vi "VeriStand Example.vi"() -> ()   [LabVIEW 2015]
uses:
  VeriStand FPGA Generation Wizard/Source/SubModules/FPGA Addon Speciality IO/Source/Types/PWM.Measure.Digital.Measurement.ctl
  VeriStand FPGA Generation Wizard/Source/SubModules/FPGA Addon Speciality IO/Source/Types/PWM.Generate.Digital.Settings.ctl
  VeriStand FPGA Generation Wizard/Source/SubModules/FPGA Addon Speciality IO/Source/Types/PWM.Measure.Analog.Measurement.ctl
  VeriStand FPGA Generation Wizard/Source/SubModules/FPGA Addon Speciality IO/Source/Types/PWM.Measure.Digital.Settings.ctl
  VeriStand FPGA Generation Wizard/Source/SubModules/FPGA Addon Speciality IO/Source/Types/PWM.Measure.Analog.Settings.ctl
  VeriStand FPGA Generation Wizard/Source/SubModules/FPGA Addon Speciality IO/Source/Types/Sine.Generate.Settings.ctl
  VeriStand FPGA Generation Wizard/Source/SubModules/FPGA Addon Speciality IO/Source/Types/Static.Generate.Digital.Settings.ctl
  VeriStand FPGA Generation Wizard/Source/SubModules/FPGA Addon Speciality IO/Source/Types/Static.Measure.Digital.Settings.ctl
  VeriStand FPGA Generation Wizard/Source/SubModules/FPGA Addon Speciality IO/Source/Types/Static.Measure.Digital.Measurement.ctl
  VeriStand FPGA Generation Wizard/Source/SubModules/FPGA Addon Speciality IO/Source/Types/WSS.Generate.Digital.Settings.ctl
  VeriStand FPGA Generation Wizard/Source/SubModules/FPGA Addon Speciality IO/Source/Types/QuadratureEncoder.Measure.Digital.Measurement.ctl
  VeriStand FPGA Generation Wizard/Source/SubModules/FPGA Addon Speciality IO/Source/Types/QuadratureEncoder.Measure.Digital.Settings.ctl
  <vilib>/Platform/TimedLoop/XDataNode/timing_clust.ctl
  <vilib>/Platform/TimedLoop/XDataNode/nitl_modes.ctl
  <vilib>/Platform/TimedLoop/XDataNode/wakeup.ctl
  <vilib>/rvi/Emulation/niFpgaGetClockAttributes.vi
  <vilib>/rvi/Emulation/niFpgaSctlEmulationGetInTimedLoop.vi
  <vilib>/rvi/Emulation/niFpgaEmulationReportErrorSimple.vi
  <vilib>/rvi/Emulation/niFpgaCriticalErrorInLSC.vi
  <vilib>/Platform/TimedLoop/XDataNode/XDataNode.xnode
  VeriStand FPGA Generation Wizard/Source/SubModules/FPGA Addon Speciality IO/Source/Speciality FPGA IO.lvlib
  <vilib>/Platform/TimedLoop/XDataNode/XDNodeRunTimeDep.lvlib
panel:
  in  "Measure.Digital.Ch5.QuadEncoder.Settings":T1={"DIRECTION"=0, "RESET VALUE"=0, "A RESET STATE"=TRUE, "B RESET STATE"=TRUE, "Z RESET STATE"=TRUE}
  in  "Z":bool
  in  "B":bool
  in  "A":bool
  out "Measurement.Digital.Ch5":T2
  out "Bit1":bool
  out "Bit0":bool
  in  "Generate.Digital.Ch4.WSS.Settings":T3={"ACTIVE EDGE"=TRUE, "ACTIVE TICKS"=0, "INACTIVE TICKS"=0, "DATA"=0, "SENSOR TYPE"=0}
  in  "Generate.Digital.Ch3.Internal.Settings":T4={"ACTIVE EDGE"=TRUE, "OUTPUT"=FALSE}
  in  "Measure.Digital.Ch3.Internal.Settings":T5={"ACTIVE EDGE"=TRUE}
  out "Measure.Digital.Ch3":T6
  out "Measure.Digital.Ch2":T6
  in  "Measure.Digital.Ch2.Internal.Settings":T5={"ACTIVE EDGE"=TRUE}
  in  "Generate.Digital.Ch2.Internal.Settings":T4={"ACTIVE EDGE"=TRUE, "OUTPUT"=FALSE}
  out "Analog.Generation.Ticks":u32=10 caption="Count(uSec)"
  in  "Generate.Sine.Ch1.Settings":T7
  in  "Generate.Sine.Ch0.Settings":T7
  in  "Sine":bool=TRUE
  in  "Measure.Analog.Ch1.Settings":T8={"ACTIVE EDGE"=FALSE, "TIMEOUT"=40000000, "THRESHOLD"=95.0}
  in  "Measure.Analog.Ch0.Settings":T8={"ACTIVE EDGE"=TRUE, "TIMEOUT"=40000000, "THRESHOLD"=0.0}
  in  "Measure.Digital.Ch1.Settings":T9={"ACTIVE EDGE"=FALSE, "TIMEOUT"=40000000}
  in  "Measure.Digital.Ch0.Settings":T9={"ACTIVE EDGE"=TRUE, "TIMEOUT"=40000000}
  out "Measure.Analog.Ch1":T10={"ACTIVE TICKS"=90, "INACTIVE TICKS"=10, "ACQ TICKS"=400, "ACTIVE VOLTAGE"=-6.998723030090332, "INACTIVE VOLTAGE"=6.998509407043457}
  out "Measure.Analog.Ch0":T10={"ACTIVE TICKS"=10, "INACTIVE TICKS"=10, "ACQ TICKS"=400, "ACTIVE VOLTAGE"=4.979251861572266, "INACTIVE VOLTAGE"=-4.979404449462891}
  in  "Generate.Digital.Ch1.Internal.Settings":T11={"ACTIVE EDGE"=FALSE, "ACTIVE TICKS"=60000000, "INACTIVE TICKS"=20000000}
  in  "Generate.Digital.Ch0.Internal.Settings":T11={"ACTIVE EDGE"=TRUE, "ACTIVE TICKS"=4000, "INACTIVE TICKS"=12000}
  out "Measure.Digital.Ch1":T12
  out "Measure.Digital.Ch0":T12={"ACTIVE TICKS"=4000, "INACTIVE TICKS"=12000, "ACQ TICKS"=1}
  in  "Analog.Generation.Ticks":u32=10 caption="Count(uSec)"
  # "98"
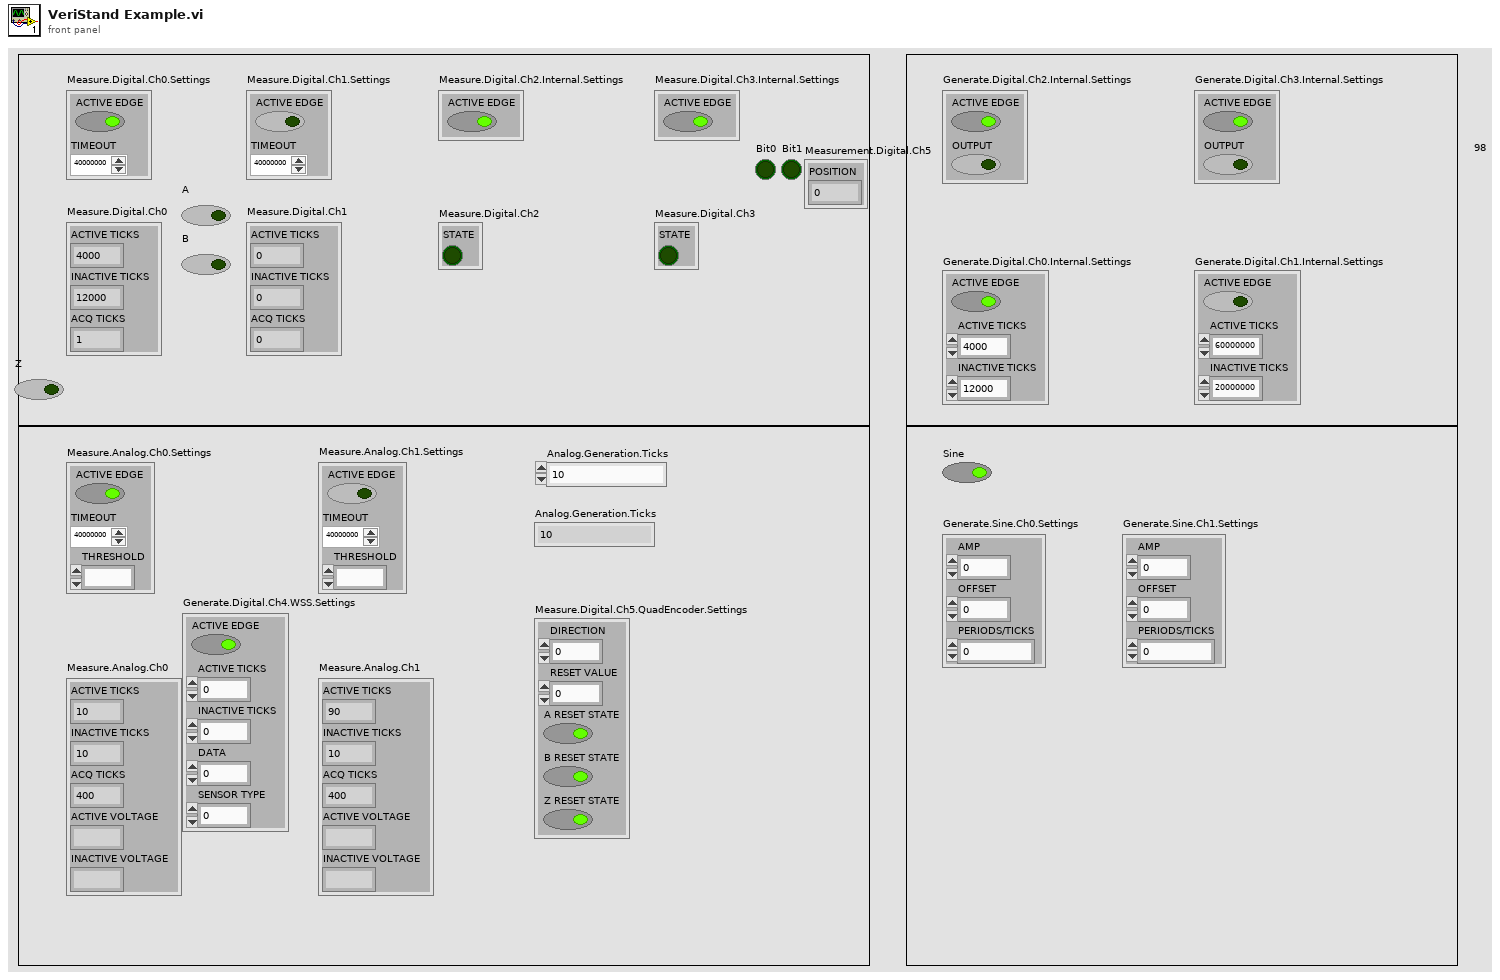
[diagram p1: front panel]
types:
  T1 = typedef "QuadratureEncoder.Measure.Digital.Settings.ctl" = cluster{"DIRECTION":u8, "RESET VALUE":i32, "A RESET STATE":bool, "B RESET STATE":bool, "Z RESET STATE":bool}
  T2 = typedef "QuadratureEncoder.Measure.Digital.Measurement.ctl" = cluster{"POSITION":i32}
  T3 = typedef "Speciality FPGA IO.lvlib/WSS.Generate.Digital.Settings.ctl" = cluster{"ACTIVE EDGE":bool, "ACTIVE TICKS":u32, "INACTIVE TICKS":u32, "DATA":u8, "SENSOR TYPE":u8}
  T4 = typedef "Speciality FPGA IO.lvlib/Static.Generate.Digital.Settings.ctl" = cluster{"ACTIVE EDGE":bool, "OUTPUT":bool}
  T5 = typedef "Speciality FPGA IO.lvlib/Static.Measure.Digital.Settings.ctl" = cluster{"ACTIVE EDGE":bool}
  T6 = typedef "Speciality FPGA IO.lvlib/Static.Measure.Digital.Measurement.ctl" = cluster{"STATE":bool}
  T7 = typedef "Speciality FPGA IO.lvlib/Sine.Generate.Settings.ctl" = cluster{"AMP":fxp<+/-,32,8>, "OFFSET":fxp<+/-,32,8>, "PERIODS/TICKS":fxp<+,32,0>}
  T8 = typedef "Speciality FPGA IO.lvlib/PWM.Measure.Analog.Settings.ctl" = cluster{"ACTIVE EDGE":bool, "TIMEOUT":u32, "THRESHOLD":fxp<+/-,32,8>}
  T9 = typedef "Speciality FPGA IO.lvlib/PWM.Measure.Digital.Settings.ctl" = cluster{"ACTIVE EDGE":bool, "TIMEOUT":u32}
  T10 = typedef "Speciality FPGA IO.lvlib/PWM.Measure.Analog.Measurement.ctl" = cluster{"ACTIVE TICKS":u32, "INACTIVE TICKS":u32, "ACQ TICKS":u32, "ACTIVE VOLTAGE":fxp<+/-,32,8>, "INACTIVE VOLTAGE":fxp<+/-,32,8>}
  T11 = typedef "Speciality FPGA IO.lvlib/PWM.Generate.Digital.Settings.ctl" = cluster{"ACTIVE EDGE":bool, "ACTIVE TICKS":u32, "INACTIVE TICKS":u32}
  T12 = typedef "Speciality FPGA IO.lvlib/PWM.Measure.Digital.Measurement.ctl" = cluster{"ACTIVE TICKS":u32, "INACTIVE TICKS":u32, "ACQ TICKS":u32}
  T13 = typedef "XDNodeRunTimeDep.lvlib/timing_clust.ctl" = cluster{"Expected End [f-1]":u64, "Actual End [f-1]":u64, "Finished Late? [f-1]":bool, "Expected End [i-1]":u64, "Actual End [i-1]":u64, "Finished Late? [i-1]":bool, "Expected Start [i]":u64, "Actual Start [i]":u64, "Expected Start [f]":u64, "Actual Start [f]":u64, "Source Name":string, "Structure Name":string, "Period":i64, "Deadline":i64, "Offset":i64, "Start":i64, "Priority":i32, "Timeout":i32, "Mode":T14, "Wakeup Reason":T15, "Error":errorcluster, "Source Type":string, "Secondary Source Type":string, "Global End Time":u64, "Global Start Time":u64, "Frame Duration":u64, "Iteration Duration":u64, "Assigned CPU":i32, "I/O Scan Engine Mode":u32}
  T14 = typedef "XDNodeRunTimeDep.lvlib/nitl_modes.ctl" = enum32{"No Change", "Process missed periods, maintain original phase", "Discard missed periods, maintain original phase", "Process missed periods, ignore original phase", "Discard missed periods, ignore original phase"}
  T15 = typedef "XDNodeRunTimeDep.lvlib/wakeup.ctl" = enum32{"Normal", "Aborted", "Asynchronous wakeup", "Timing source error", "Timed loop error", "Timeout"}
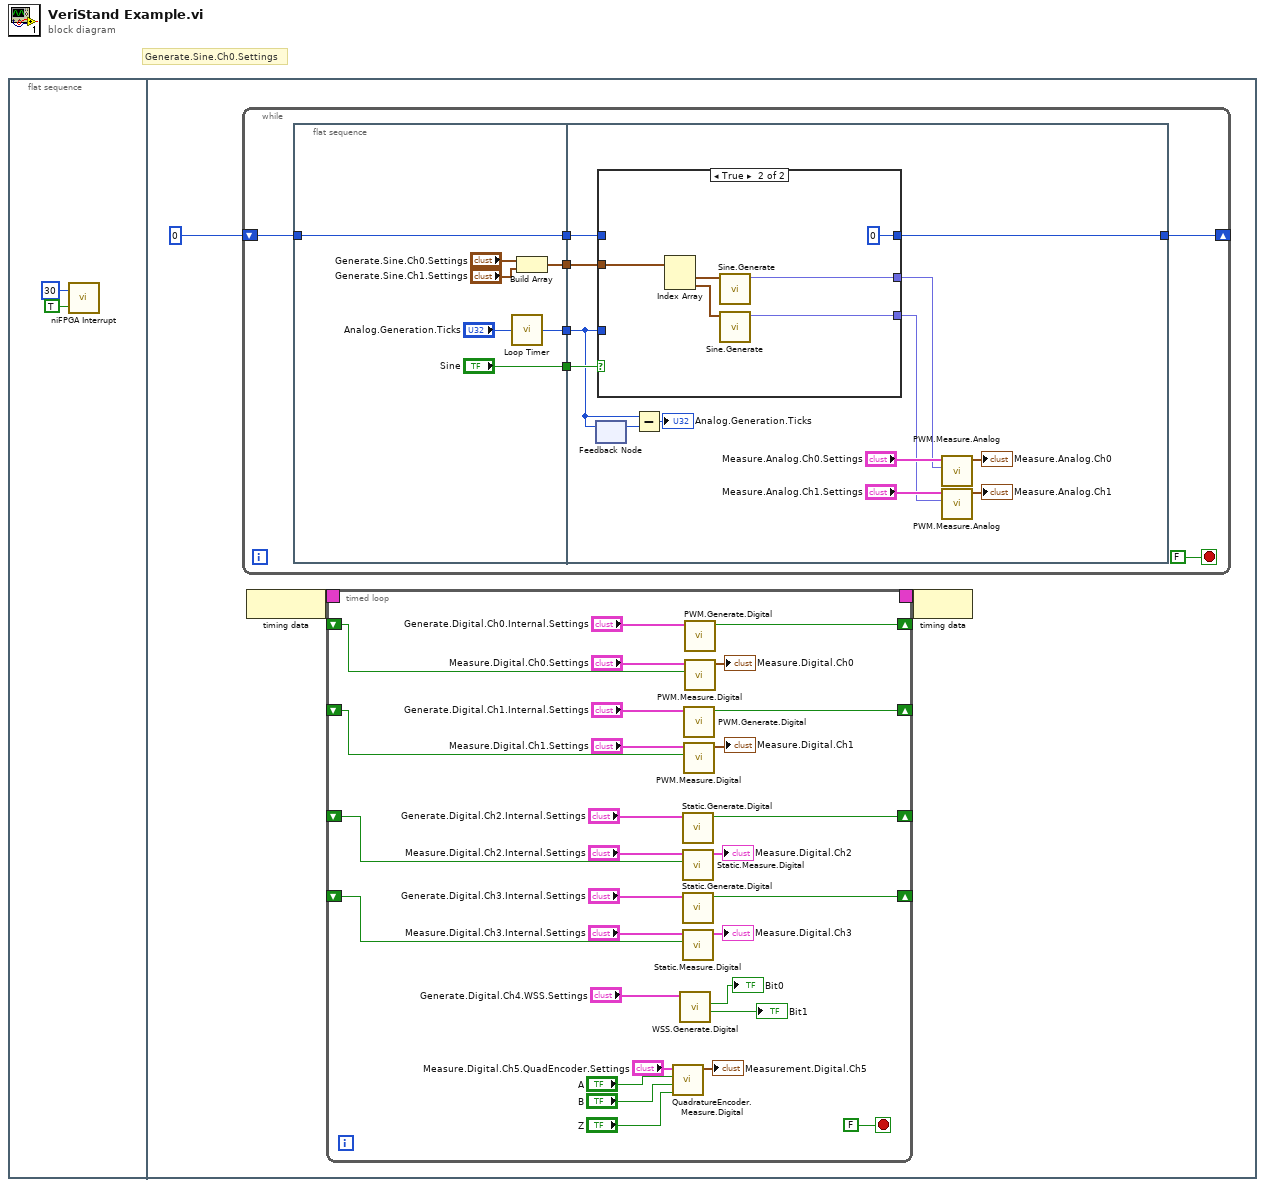
[diagram p0: block diagram]
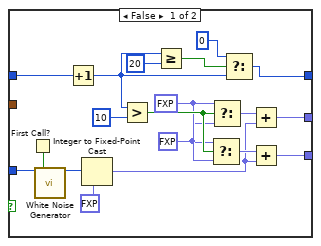
[diagram p2: hidden frame]
diagram:
  # "Generate.Sine.Ch0.Settings"
  n1 = flat-sequence {
    frame #0 {
      n2 = call <vilib>:"niFPGA Interrupt.vi"("Wait Until Cleared (F)"=TRUE, "IRQ Number (0)"=u8 30) -> ()  [unwired: 1 in]
    }
    frame #1 {
      n3 = while {
        shift-right: [w43] -> _
        shift-left: i16 0 -> [w44]
        stop <- FALSE stop-if-true
        n4 = flat-sequence {
          tunnel: [w51] -> w45
          tunnel: w44 -> [w51]
          tunnel: [w50] -> w42
          tunnel: ["Sine"] -> w40
          tunnel: [w46] -> w39
          tunnel: w45 -> [w58]
          tunnel: [w59] -> w43
          tunnel: w42 -> [w54]
          tunnel: w40 -> [w57]
          tunnel: w39 -> [w56]
          frame #0 {
            n5 = call "Loop Timer"("Count(uSec)"="Analog.Generation.Ticks") -> ("Tick Count(uSec)"=w50:u32)
            n6 = Build Array("Generate.Sine.Ch0.Settings", "Generate.Sine.Ch1.Settings") -> (w46:T7[])
          }
          frame #1 {
            n7 = feedback-in #1(w54) -> ()
            n8 = feedback #1() -> (w55:u32)  [unwired: 1 in]
            n9 = case shown="True" w57 {
              tunnel: [w67 w85] -> w61
              tunnel: [w68 w86] -> w60
              tunnel: w58 -> [w71 _]
              tunnel: w54 -> [w70 _]
              tunnel: [w69 i16 0 ("t")] -> w59
              tunnel: w56 -> [_ w89]
              frame False {
                w78 = fxp<+/-,32,8> 12.0 ("t")
                w79 = fxp<+/-,32,8> -12.0 ("PWM")
                n10 = First Call?() -> (First Call?: T/F=w77:bool)
                n11 = call "White Noise Generator"("seed"=w70, "reset"=w77) -> ("white noise out"=w76:i16)  [unwired: 13 in]
                n12 = Increment(x=w71) -> (x+1=w81:i16)
                n13 = Integer to Fixed-Point Cast(fixed-point type=fxp<+/-,16,1> 0.0, integer=w76) -> (fixed-point=w66:fxp<+/-,16,1>)
                n14 = Greater?(x=w81, y=i16 10) -> (0:w80:bool)
                n15 = Greater Or Equal?(x=w81, y=i16 20) -> (x >= y?=w72:bool)
                n16 = Select(t=w78, s=w80, f=w79) -> (s? t:f=w73:fxp<+/-,32,8>)
                n17 = Select(t=w79, s=w80, f=w78) -> (s? t:f=w74:fxp<+/-,32,8>)
                n18 = Select(t=i16 0, s=w72, f=w81) -> (s? t:f=w69:i16)
                n19 = Add(x=w74, y=w66) -> (x+y=w68:fxp<+/-,33,9>)
                n20 = Add(x=w73, y=w66) -> (x+y=w67:fxp<+/-,33,9>)
              }
              frame True {
                n21 = Index Array(array=w89) -> (element #1=w88:T7, element #2=w87:T7)  [unwired: 2 in]
                n22 = call "Sine.Generate.vi"("Settings"=w88) -> ("Output"=w86:fxp<+/-,32,8>)  [unwired: 10 in]
                n23 = call "Sine.Generate.vi"("Settings"=w87) -> ("Output"=w85:fxp<+/-,32,8>)  [unwired: 10 in]
              }
            }
            n24 = Subtract(x=w54, y=w55) -> (x-y=→"Analog.Generation.Ticks":u32)
            n25 = call "PWM.Measure.Analog.vi"("PWM"=w60, "Settings"="Measure.Analog.Ch0.Settings") -> ("Measurement"=→"Measure.Analog.Ch0":T10)  [unwired: 8 in, 1 out]
            n26 = call "PWM.Measure.Analog.vi"("PWM"=w61, "Settings"="Measure.Analog.Ch1.Settings") -> ("Measurement"=→"Measure.Analog.Ch1":T10)  [unwired: 8 in, 1 out]
          }
        }
      }
      n27 = node-c288() -> (w5:T13)
      n28 = timed-loop {
        timing: w5 -> [_]
        timing-out: [_] -> w4
        shift-right: [w33] -> _
        shift-left: _ -> [w32]
        shift-right: [w31] -> _
        shift-left: _ -> [w30]
        shift-right: [w23] -> _
        shift-left: _ -> [w21]
        shift-right: [w14] -> _
        shift-left: _ -> [w16]
        stop <- FALSE stop-if-true
        n29 = call "QuadratureEncoder.Measure.Digital.vi"("Z"="Z", "B"="B", "A"="A", "Settings"="Measure.Digital.Ch5.QuadEncoder.Settings") -> ("Measurement"=→"Measurement.Digital.Ch5":T2)  [unwired: 7 in]
        n30 = call "WSS.Generate.Digital.vi"("Settings"="Generate.Digital.Ch4.WSS.Settings") -> ("Bit1"=→"Bit1":bool, "Bit0"=→"Bit0":bool)  [unwired: 9 in]
        n31 = call "Static.Generate.Digital.vi"("Settings"="Generate.Digital.Ch2.Internal.Settings") -> ("Output"=w23:bool)  [unwired: 10 in]
        n32 = call "Static.Measure.Digital.vi"("State"=w21, "Settings"="Measure.Digital.Ch2.Internal.Settings") -> ("Measurement"=→"Measure.Digital.Ch2":T6)  [unwired: 9 in]
        n33 = call "Static.Generate.Digital.vi"("Settings"="Generate.Digital.Ch3.Internal.Settings") -> ("Output"=w14:bool)  [unwired: 10 in]
        n34 = call "Static.Measure.Digital.vi"("State"=w16, "Settings"="Measure.Digital.Ch3.Internal.Settings") -> ("Measurement"=→"Measure.Digital.Ch3":T6)  [unwired: 9 in]
        n35 = call "PWM.Generate.Digital.vi"("Settings"="Generate.Digital.Ch1.Internal.Settings") -> ("Output"=w33:bool)  [unwired: 10 in]
        n36 = call "PWM.Measure.Digital.vi"("State"=w32, "Settings"="Measure.Digital.Ch1.Settings") -> ("Measurement"=→"Measure.Digital.Ch1":T12)  [unwired: 8 in, 1 out]
        n37 = call "PWM.Generate.Digital.vi"("Settings"="Generate.Digital.Ch0.Internal.Settings") -> ("Output"=w31:bool)  [unwired: 10 in]
        n38 = call "PWM.Measure.Digital.vi"("State"=w30, "Settings"="Measure.Digital.Ch0.Settings") -> ("Measurement"=→"Measure.Digital.Ch0":T12)  [unwired: 8 in, 1 out]
      }
      n39 = node-c288(w4) -> ()
    }
  }
